vi "Teleop.vi"(10 "Match Info":T1={"Autonomous Elapsed Seconds"=0.0, "TeleOp Elapsed Seconds"=0.0, "Disabled Elapsed Seconds"=0.0, "Visited Autonomous"=FALSE, "Visited TeleOp"=FALSE, "Visited Disabled"=FALSE, "Autonomous Settings"={"Autonomous Style"=enum."Independent", "VI Refnum"=refnum}}, 11 "Call Context":T2) -> ()   [LabVIEW 2017]
doc: "This VI is called for each enabled TeleOp packet received from the DS. It is typically used to read from joysticks and other inputs and update I/O or setpoints for timed control loops. It should complete and return within 20 milliseconds or risk missing DS packets."
uses:
  <vilib>/Rock Robotics/WPI/DriverStation/WPI_DriverStationDerivedRobotMode.ctl
  <vilib>/Rock Robotics/WPI/DriverStation/WPI_DriverStationMatch Info.ctl
  <vilib>/Rock Robotics/WPI/Utilities/WPI_GetSetVariantRefNum.vi
  <vilib>/Rock Robotics/WPI/RobotDrive/WPI_RobotDriveMecanumDrive_Cartesian.vi
  <vilib>/Rock Robotics/WPI/Solenoid/WPI_SolenoidValue.ctl
  <vilib>/Rock Robotics/WPI/Solenoid/WPI_SolenoidSetEnum.vi
panel:
  out "Distance":dbl
  out "Magnet sensed 2":bool
  out "Magnet sensed 1":bool
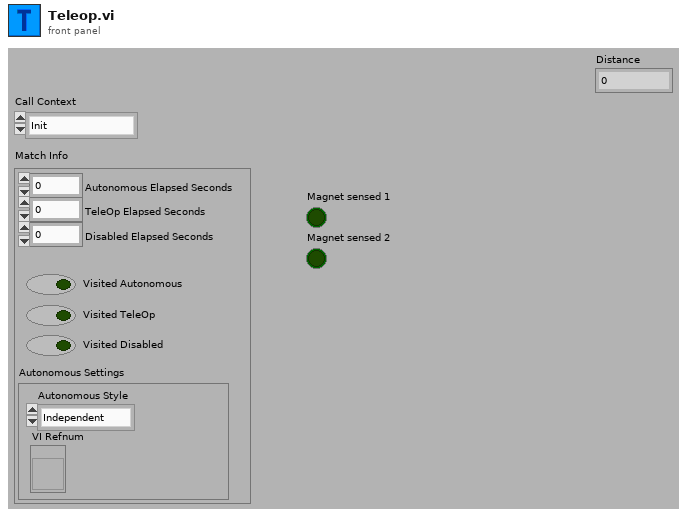
[diagram p1: front panel]
types:
  T1 = typedef "WPI_DriverStationMatch Info.ctl" = cluster{"Autonomous Elapsed Seconds":dbl, "TeleOp Elapsed Seconds":dbl, "Disabled Elapsed Seconds":dbl, "Visited Autonomous":bool, "Visited TeleOp":bool, "Visited Disabled":bool, "Autonomous Settings":cluster{"Autonomous Style":enum16{"Iterative", "Independent"}, "VI Refnum":refnum<vi>}}
  T2 = typedef "WPI_DriverStationDerivedRobotMode.ctl" = enum16{"Init", "Execute", "Stop"}
  T3 = typedef "WPI_SolenoidValue.ctl" = enum16{"Off", "On", "Forward", "Reverse"}
  T4 = typedef "WPI_DigitalInputDevRef.ctl" = cluster{"DevStatus":errorcluster, "DIO Channel":T5}
  T5 = typedef "FPGA_DIOChannel.ctl" = enum8{"DIO 0", "DIO 1", "DIO 2", "DIO 3", "DIO 4", "DIO 5", "DIO 6", "DIO 7", "DIO 8", "DIO 9", "DIO MXP 0", "DIO MXP 1", "DIO MXP 2", "DIO MXP 3", "DIO MXP 4", "DIO MXP 5", "DIO MXP 6", "DIO MXP 7", "DIO MXP 8", "DIO MXP 9", "DIO MXP 10", "DIO MXP 11", "DIO MXP 12", "DIO MXP 13", "DIO MXP 14", "DIO MXP 15", "SPI Port CS1", "SPI Port CS2", "SPI Port CS3", "SPI Port MISO", "SPI Port MOSI", "Invalid"}
  T6 = typedef "WPI_SolenoidDevRef.ctl" = cluster{"DevStatus":errorcluster, "Pneumatics Control Module":u8, "Forward Solenoid Channel":T7, "Reverse Solenoid Channel":T7}
  T7 = typedef "WPI_SolenoidChannel.ctl" = enum8{"Solenoid 0", "Solenoid 1", "Solenoid 2", "Solenoid 3", "Solenoid 4", "Solenoid 5", "Solenoid 6", "Solenoid 7", "Invalid"}
  T8 = typedef "WPI_CompressorDevRef.ctl" = cluster{"DevStatus":errorcluster, "Pneumatics Control Module":u8}
  T9 = typedef "WPI_JoystickDevRef.ctl" = cluster{"Device":T10}
  T10 = typedef "WPI_JoystickDeviceEnum.ctl" = enum16{"USB 0", "USB 1", "USB 2", "USB 3", "USB 4", "USB 5"}
  T11 = cluster{"Buttons[0]":bool, "Buttons[1]":bool, "Buttons[2]":bool, "Buttons[3]":bool, "Buttons[4]":bool, "Buttons[5]":bool, "Buttons[6]":bool, "Buttons[7]":bool, "Buttons[8]":bool}
  T12 = cluster{"Axes[0]":dbl, "Axes[1]":dbl, "Axes[2]":dbl, "Axes[3]":dbl, "Axes[4]":dbl, "Axes[5]":dbl, "Axes[6]":dbl, "Axes[7]":dbl, "Axes[8]":dbl}
  T13 = typedef "WPI_RobotDriveDevRef.ctl" = cluster{"DevStatus":errorcluster, "Motors[]":T14[], "Square Inputs":bool, "Max Output":dbl}
  T14 = typedef "WPI_MotorControlDeviceRef.ctl" = cluster{"DeviceStatus":errorcluster, "Type":T15, "PWM":cluster{"PWM Channel":T16, "DeadBand":T17}, "CAN":cluster{"Device Number":u8, "SetOutput VI Ref":variant, "GetOutput VI Ref":variant, "Enable VI Ref":variant, "Disable VI Ref":variant, "Data":variant}, "Invert":bool, "DIO PWM":cluster{"PWM \"Enable\" Channel":T16, "DIOChannel":T5, "PWM Rate":dbl}}
  T15 = typedef "WPI_MotorControlType.ctl" = enum16{"PWM", "CAN", "DIO PWM"}
  T16 = typedef "FPGA_DIOPWMChannel.ctl" = enum8{"PWM 0", "PWM 1", "PWM 2", "PWM 3", "PWM 4", "PWM 5", "PWM 6", "PWM 7", "PWM 8", "PWM 9", "PWM MXP 0", "PWM MXP 1", "PWM MXP 2", "PWM MXP 3", "PWM MXP 4", "PWM MXP 5", "PWM MXP 6", "PWM MXP 7", "PWM MXP 8", "PWM MXP 9", "Invalid"}
  T17 = typedef "WPI_PWMDeadband.ctl" = cluster{"Name":string, "maxPositivePwm":i32, "minPositivePwm":i32, "centerPwm":i32, "maxNegativePwm":i32, "minNegativePwm":i32, "angularRange":u16}
  T18 = typedef "WPI_EncoderDevRef.ctl" = cluster{"DevStatus":errorcluster, "EncoderIndex":T19, "CounterIndex":T20, "DistancePerCount":dbl, "Decoding Type":T21}
  T19 = typedef "FPGA_EncoderIdx.ctl" = enum8{"Enc 0", "Enc 1", "Enc 2", "Enc 3", "Enc 4", "Enc 5", "Enc 6", "Enc 7", "Invalid"}
  T20 = typedef "FPGA_CounterCtrSystemIndex.ctl" = enum8{"Ctr 0", "Ctr 1", "Ctr 2", "Ctr 3", "Ctr 4", "Ctr 5", "Ctr 6", "Ctr 7", "Invalid"}
  T21 = typedef "WPI_EncoderType.ctl" = enum16{"1x", "2x", "4x"}
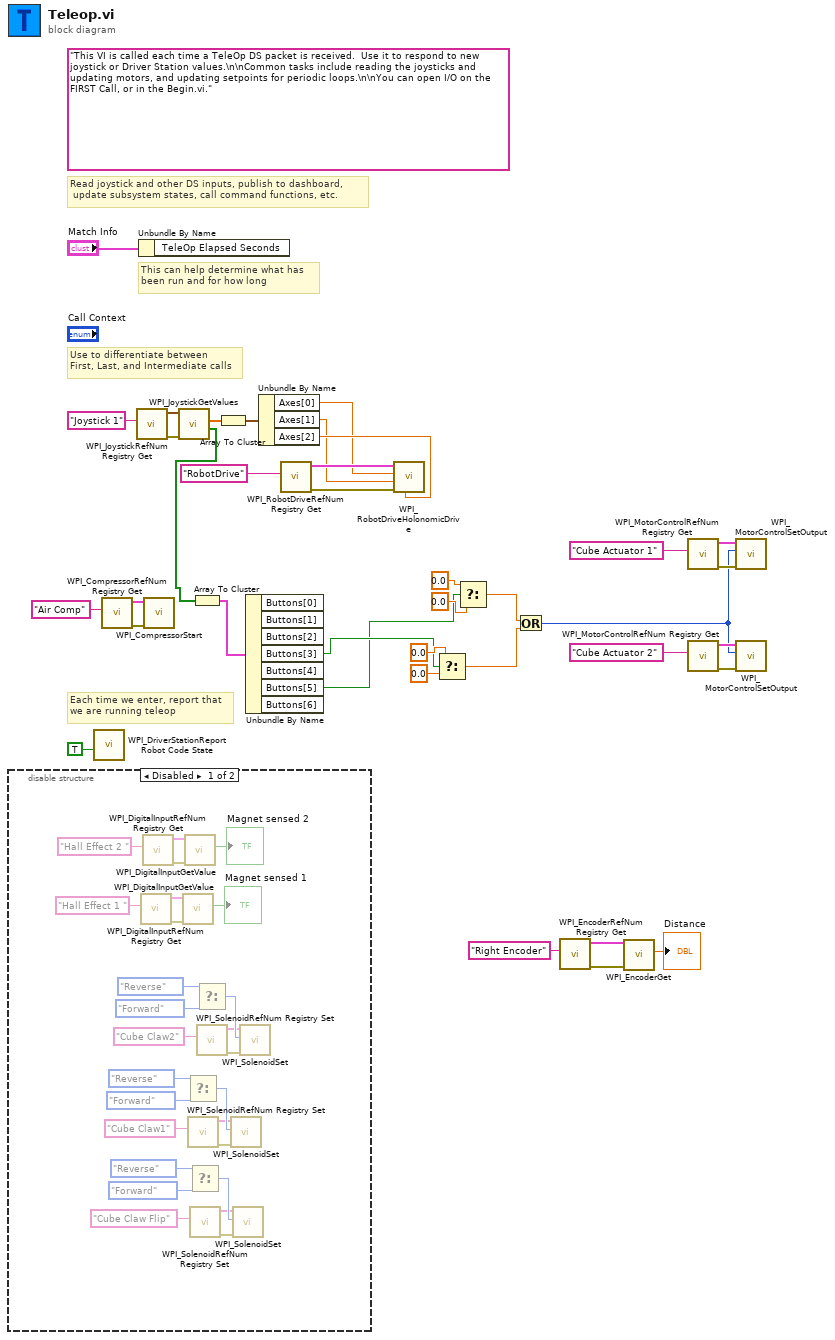
[diagram p0: block diagram]
diagram:
  (unwired) "This VI is called each time a TeleOp DS packet is received.  Use it to respond to new joystick or Driver Station values.\n\nCommon tasks include reading the joysticks and updating motors, and updating setpoints for periodic loops.\n\nYou can open I/O on the FIRST Call, or in the Begin.vi."
  # "Read joystick and other DS inputs, publish to dashboard,\n update subsystem states, call command functions, etc."
  # "Each time we enter, report that\nwe are running teleop"
  # "Use to differentiate between\nFirst, Last, and Intermediate calls"
  # "This can help determine what has\nbeen run and for how long"
  n1 = disable-structure shown="Disabled" {
    frame Disabled {
      n2 = call <vilib>:"WPI_DigitalInputRefNum Registry Get.vi"("refnum name"="Hall Effect 1 ") -> ("error out"=w42:errorcluster, "DigitalInputDevRef"=w41:T4)  [unwired: 9 in]
      n3 = call <vilib>:"WPI_DigitalInputRefNum Registry Get.vi"("refnum name"="Hall Effect 2 ") -> ("error out"=w45:errorcluster, "DigitalInputDevRef"=w44:T4)  [unwired: 9 in]
      n4 = call <vilib>:"WPI_DigitalInputGetValue.vi"("error in (no error)"=w42, "DigitalInputDevRef"=w41) -> ("Value"=→"Magnet sensed 1":bool)  [unwired: 7 in, 2 out]
      n5 = call <vilib>:"WPI_DigitalInputGetValue.vi"("error in (no error)"=w45, "DigitalInputDevRef"=w44) -> ("Value"=→"Magnet sensed 2":bool)  [unwired: 7 in, 2 out]
      n6 = Select(t=WPI_SolenoidValue."Reverse" ("Value"), f=WPI_SolenoidValue."Forward" ("Value")) -> (s? t:f=w57:T3)  [unwired: 1 in]
      n7 = call <vilib>:"WPI_SolenoidRefNum Registry Set.vi"("refnum name"="Cube Claw1") -> ("error out"=w56:errorcluster, "SolenoidDevRef"=w55:T6)  [unwired: 9 in]
      n8 = Select(t=WPI_SolenoidValue."Reverse" ("Value"), f=WPI_SolenoidValue."Forward" ("Value")) -> (s? t:f=w63:T3)  [unwired: 1 in]
      n9 = call <vilib>:"WPI_SolenoidRefNum Registry Set.vi"("refnum name"="Cube Claw Flip") -> ("error out"=w62:errorcluster, "SolenoidDevRef"=w61:T6)  [unwired: 9 in]
      n10 = Select(t=WPI_SolenoidValue."Reverse" ("Value"), f=WPI_SolenoidValue."Forward" ("Value")) -> (s? t:f=w60:T3)  [unwired: 1 in]
      n11 = call <vilib>:"WPI_SolenoidRefNum Registry Set.vi"("refnum name"="Cube Claw2") -> ("error out"=w59:errorcluster, "SolenoidDevRef"=w58:T6)  [unwired: 9 in]
      n12 = call-poly <vilib>:"WPI_SolenoidSet.vi"("error in (no error)"=w56, "Value"=w57, "SolenoidDevRef"=w55) -> ()  [unwired: 7 in, 2 out]
      n13 = call-poly <vilib>:"WPI_SolenoidSet.vi"("error in (no error)"=w62, "Value"=w63, "SolenoidDevRef"=w61) -> ()  [unwired: 7 in, 2 out]
      n14 = call-poly <vilib>:"WPI_SolenoidSet.vi"("error in (no error)"=w59, "Value"=w60, "SolenoidDevRef"=w58) -> ()  [unwired: 7 in, 2 out]
    }
    frame Enabled {
    }
  }
  n15 = call <vilib>:"WPI_DriverStationReport Robot Code State.vi"("TeleOp"=TRUE ("Autonomous")) -> ()  [unwired: 10 in, 1 out]
  n16 = call <vilib>:"WPI_CompressorRefNum Registry Get.vi"("refnum name"="Air Comp") -> ("error out"=w28:errorcluster, "CompressorDevRef"=w27:T8)  [unwired: 9 in]
  n17 = call <vilib>:"WPI_JoystickRefNum Registry Get.vi"("refnum name"="Joystick 1") -> ("error out"=w32:errorcluster, "JoystickDevRef"=w31:T9)  [unwired: 9 in]
  n18 = Unbundle By Name("Match Info") -> ()  [unwired: 1 out]
  n19 = call <vilib>:"WPI_CompressorStart.vi"("error in (no error)"=w28, "CompressorDevRef"=w27) -> ()  [unwired: 8 in, 2 out]
  n20 = call <vilib>:"WPI_JoystickGetValues.vi"("error in (no error)"=w32, "JoystickDevRef"=w31) -> ("Buttons"=w22:bool[], "Axes"=w4:dbl[])  [unwired: 5 in, 3 out]
  n21 = Array To Cluster(array=w22) -> (cluster=w21:T11)
  n22 = Array To Cluster(array=w4) -> (cluster=w5:T12)
  n23 = Unbundle By Name(w21) -> ("Buttons[3]"=w8:bool, "Buttons[5]"=w7:bool)  [unwired: 5 out]
  n24 = Unbundle By Name(w5) -> ("Axes[0]"=w1:dbl, "Axes[1]"=w2:dbl, "Axes[2]"=w3:dbl)
  n25 = call <vilib>:"WPI_RobotDriveRefNum Registry Get.vi"("refnum name"="RobotDrive") -> ("error out"=w33:errorcluster, "RobotDriveDevRef"=w34:T13)  [unwired: 9 in]
  n26 = call-poly <vilib>:"WPI_RobotDriveHolonomicDrive.vi"("Rotation"=w3, "error in (no error)"=w33, "Y"=w2, "X"=w1, "RobotDriveDevRef"=w34) -> ()  [unwired: 4 in, 3 out]
  n27 = Select(t=0.0, s=w8, f=0.0) -> (s? t:f=w10:dbl)
  n28 = Select(t=0.0, s=w7, f=0.0) -> (s? t:f=w9:dbl)
  n29 = Or(x=w9, y=w10) -> (x .or. y?=w6:i32)
  n30 = call <vilib>:"WPI_EncoderRefNum Registry Get.vi"("refnum name"="Right Encoder") -> ("error out"=w25:errorcluster, "EncoderDevRef"=w26:T18)  [unwired: 9 in]
  n31 = call <vilib>:"WPI_EncoderGet.vi"("error in (no error)"=w25, "EncoderDevRef"=w26) -> ("Distance"=→"Distance":dbl)  [unwired: 4 in, 5 out]
  n32 = call <vilib>:"WPI_MotorControlRefNum Registry Get.vi"("refnum name"="Cube Actuator 1") -> ("error out"=w18:errorcluster, "MotorControlDevRef"=w13:T14)  [unwired: 9 in]
  n33 = call <vilib>:"WPI_MotorControlRefNum Registry Get.vi"("refnum name"="Cube Actuator 2") -> ("error out"=w20:errorcluster, "MotorControlDevRef"=w19:T14)  [unwired: 9 in]
  n34 = call <vilib>:"WPI_MotorControlSetOutput.vi"("error in (no error)"=w18, "Output"=w6, "MotorControlDevRef"=w13) -> ()  [unwired: 6 in, 3 out]
  n35 = call <vilib>:"WPI_MotorControlSetOutput.vi"("error in (no error)"=w20, "Output"=w6, "MotorControlDevRef"=w19) -> ()  [unwired: 6 in, 3 out]
